vi "GetPosReg.vi"(10 "Ftp":refnum<k24>, 11 "error in":errorcluster) -> (2 "PosReg":T1(array[cluster]), 3 "error out":errorcluster)   [LabVIEW 2020, in "UnderAutomation.Fanuc.lvlib"]
uses:
  UnderAutomation.Fanuc.lvlib
  C:/Users/fg/Documents/Fanuc.vi/LabVIEW_2024/UnderAutomation.Fanuc/lib/UnderAutomation.Fanuc.dll
  LabVIEW_2024/UnderAutomation.Fanuc/lib/UnderAutomation.Fanuc.dll
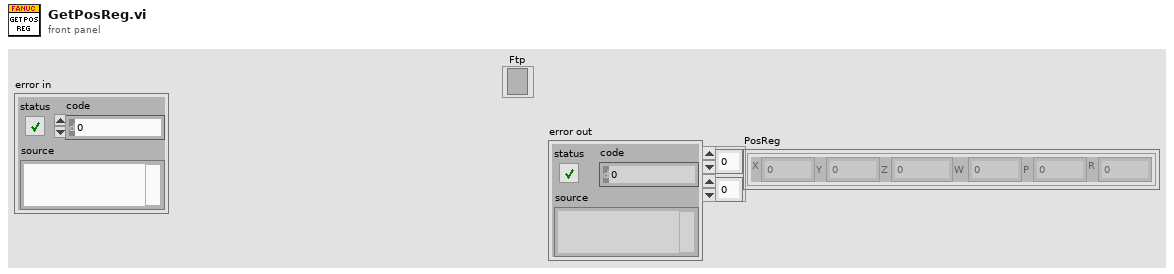
[diagram p1: front panel]
types:
  T1 = cluster{"X":dbl, "Y":dbl, "Z":dbl, "W":dbl, "P":dbl, "R":dbl}[][]
  T2 = cluster{"X":dbl, "Y":dbl, "Z":dbl, "W":dbl, "P":dbl, "R":dbl}
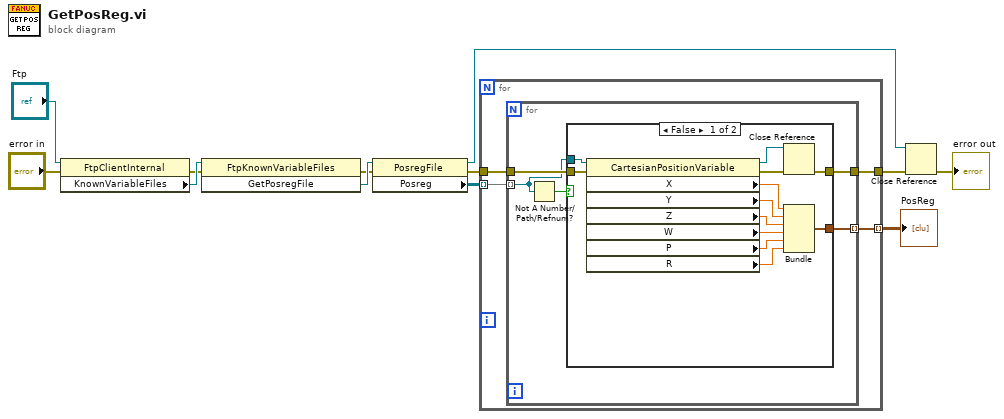
[diagram p0: block diagram]
diagram:
  n1 = property class="FtpClientInternal"(reference="Ftp", error in="error in") -> (error out=w10:errorcluster, "KnownVariableFiles"=w11:refnum<k24>)  [unwired: 1 out]
  n2 = invoke class="FtpKnownVariableFiles" method="GetPosregFile"(reference=w11, error in=w10) -> (error out=w1:errorcluster, "GetPosregFile"=w8:refnum<k24>)  [unwired: 1 in, 1 out]
  n3 = property class="PosregFile"(reference=w8, error in=w1) -> (reference out=w3:refnum<k24>, error out=w2:errorcluster, "Posreg"=w7:refnum<k24>[][])
  n4 = for {
    tunnel: w7 -> [w16] mode=indexing
    tunnel: [w15] -> w6 mode=indexing
    tunnel: w2 -> [w14]
    tunnel: [w13] -> w5
    n5 = for {
      tunnel: w16 -> [w18] mode=indexing
      tunnel: [w21] -> w15 mode=indexing
      tunnel: w14 -> [w20]
      tunnel: [w19] -> w13
      n6 = Not A Number/Path/Refnum?(number/path/refnum=w18) -> (NaN/Path/Refnum?=w17:bool)
      n7 = case shown="False" w17 {
        tunnel: [w29 _] -> w21
        tunnel: w20 -> [w28 w34]
        tunnel: [w23 w34] -> w19
        tunnel: w18 -> [w25 _]
        frame False {
          n8 = property class="CartesianPositionVariable"(reference=w25, error in=w28) -> (reference out=w22:refnum<k24>, error out=w24:errorcluster, "X"=w27:dbl, "Y"=w26:dbl, "Z"=w33:dbl, "W"=w32:dbl, "P"=w31:dbl, "R"=w30:dbl)
          n9 = Close Reference(reference=w22, error in (no error)=w24) -> (error out=w23:errorcluster)
          n10 = Bundle("X"=w27, "Y"=w26, "Z"=w33, "W"=w32, "P"=w31, "R"=w30) -> (w29:T2)  [unwired: 1 in]
        }
        frame True {
        }
      }
    }
  }
  "PosReg" <- w6
  n11 = Close Reference(reference=w3, error in (no error)=w5) -> (error out=→"error out":errorcluster)
